vi "Compile Directional Speed 1.0 Data.vi"(8 "error in (no error)":errorcluster, 11 "Device Item Ref in":T3 format="%.0x") -> (0 "error out":errorcluster, 1 "bitfile names":string[](array[string]), 2 "Directional Speeds":T1[](array[typedef]), 3 "Device Item Ref out":T3 format="%.0x")   [LabVIEW 2015, in "Engine Simulation Toolkit System Explorer.lvlib"]
uses:
  Engine Simulation Toolkit System Explorer.lvlib
  <vilib>/NI Veristand/Custom Device API/Custom Device Item Ref.ctl
  Shared/1.0 Directional Speed Engine Data.ctl
  Shared/1.0 Directional Speed FIFO Idxs.ctl
  Digital Pattern Find Events Enum.ctl
  Custom wrapped 10 bit counter.vi
  Shared/Constants and GUIDs.vi
  <vilib>/NI Veristand/Custom Device Tools/Custom Device Utility Library/NI VeriStand - Search for All Items by GUID.vi
  Shared/Properties.vi
  <vilib>/NI Veristand/Custom Device API/Get Item Property (String).vi
  <vilib>/NI Veristand/Custom Device API/Get Item Property (Dependent Node Pointer).vi
  <vilib>/NI Veristand/Custom Device Tools/Custom Device Utility Library/Custom Device Utility Library.lvlib
  Shared/Engine Simulation Toolkit Shared.lvlib
  <vilib>/NI Veristand/Custom Device API/Custom Device API.lvlib
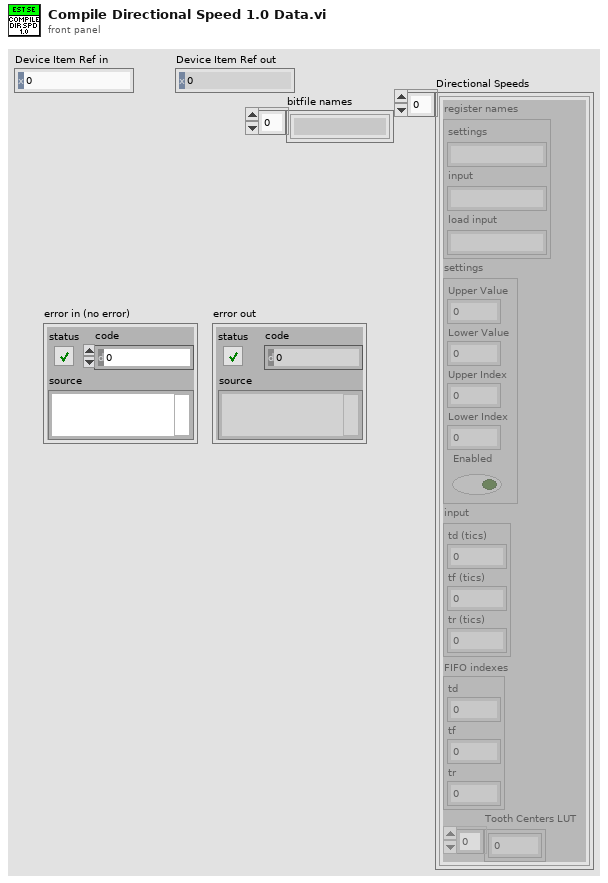
[diagram p1: front panel]
types:
  T1 = typedef "Engine Simulation Toolkit Shared.lvlib/1.0 Directional Speed Engine Data.ctl" = cluster{"register names":cluster{"settings":string, "input":string, "load input":string}, "settings":cluster{"Upper Value":u16, "Lower Value":u16, "Upper Index":fxp<+,10,10>, "Lower Index":fxp<+,10,10>, "Enabled":bool}, "input":cluster{"td (tics)":u16, "tf (tics)":u16, "tr (tics)":u16}, "FIFO indexes":T2, "Tooth Centers LUT":u16[]}
  T2 = typedef "Engine Simulation Toolkit Shared.lvlib/1.0 Directional Speed FIFO Idxs.ctl" = cluster{"td":i32, "tf":i32, "tr":i32}
  T3 = typedef "Custom Device API.lvlib/Custom Device Item Ref.ctl" = u64
  T4 = typedef "Engine Simulation Toolkit Shared.lvlib/Channel.ctl" = cluster{"Name":string, "Units":string, "Default":dbl, "Description":string}
  T5 = typedef "Engine Simulation Toolkit System Explorer.lvlib/Digital Pattern Find Events Enum.ctl" = enum16{"Rising Edge", "Falling Edge", "Any Edge", "Center Tooth", "Center Gap"}
  T6 = typedef "Custom Device API.lvlib/Custom Device Item Info.ctl" = cluster{"Name":string, "Is Channel":bool, "GUID":string, "Is Waveform":bool}
  T7 = typedef "Engine Simulation Toolkit System Explorer.lvlib/Digital Pattern.ctl" = cluster{"Name":string, "Base":T8, "Remove":T9[], "Add":T10[], "FPGA Resource":string}
  T8 = typedef "Engine Simulation Toolkit System Explorer.lvlib/Digital Pattern Base.ctl" = cluster{"Length":dbl, "Teeth":u16, "Width":dbl, "Offset":dbl}
  T9 = typedef "Engine Simulation Toolkit System Explorer.lvlib/Digital Pattern Remove Edge.ctl" = cluster{"Tooth":u16, "Edge":bool}
  T10 = typedef "Engine Simulation Toolkit System Explorer.lvlib/Digital Pattern Add Pulse.ctl" = cluster{"Tooth":u16, "Offset":dbl, "Width":dbl}
  T11 = typedef "Engine Simulation Toolkit System Explorer.lvlib/Digital Pattern Expanded.ctl" = cluster{"X":dbl[], "Y":dbl[]}
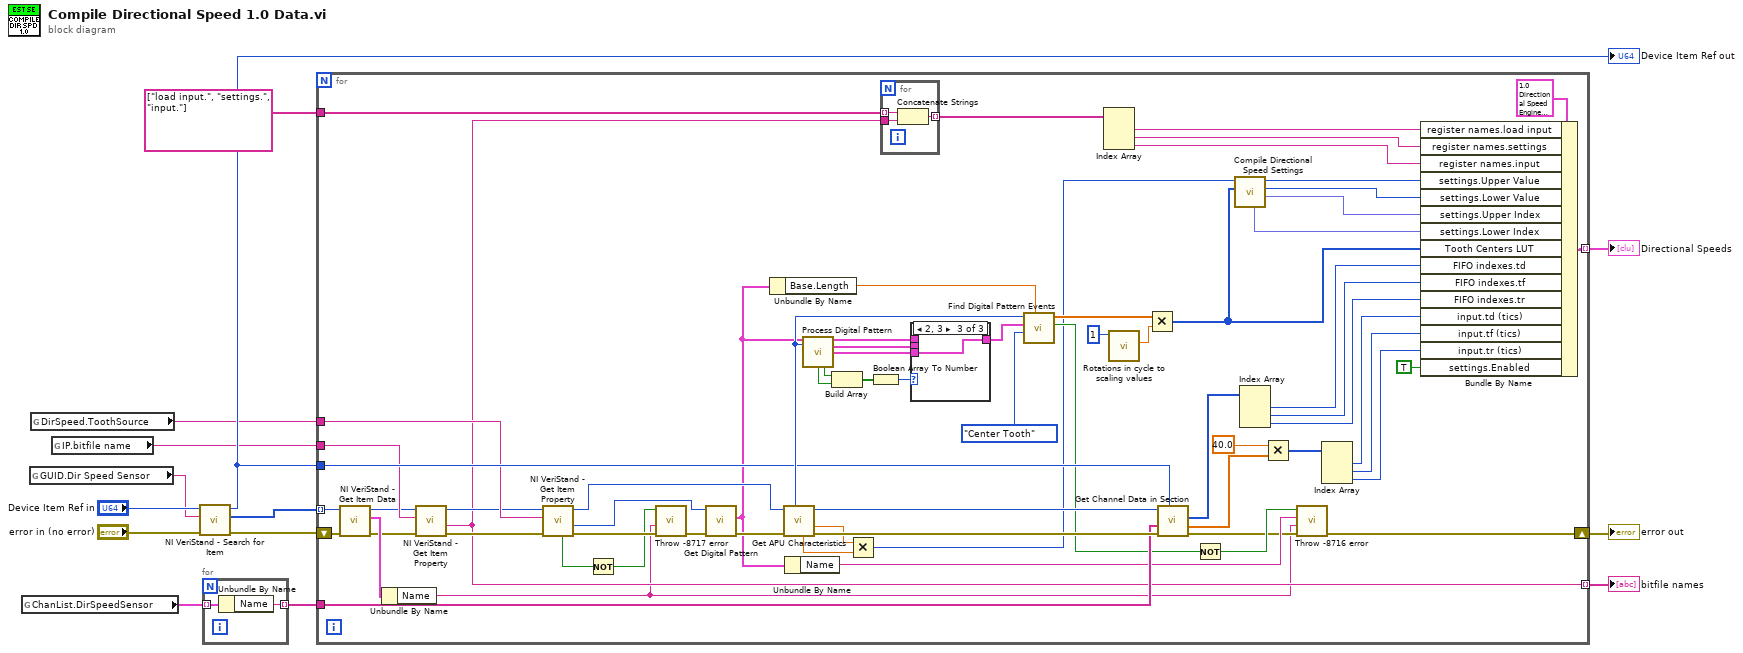
[diagram p0: block diagram]
diagram:
  n1 = global read "Constants and GUIDs.vi" "ChanList.DirSpeedSensor"() -> (w6:T4[])
  n2 = global read "Constants and GUIDs.vi" "GUID.Dir Speed Sensor"() -> (w12:string)
  n3 = global read "Properties.vi" "DirSpeed.ToothSource"() -> (w4:string)
  n4 = global read "Properties.vi" "IP.bitfile name"() -> (w3:string)
  n5 = call-poly <vilib>:"NI VeriStand - Search for Item.vi"("error in"="error in (no error)", "Item GUID"=w12, "Section Ref in"="Device Item Ref in") -> ("error out"=w11:errorcluster, "Item Refs"=w7:T3[], "Section Ref out"=w8:T3)  [unwired: 5 in, 1 out]
  "Device Item Ref out" <- w8
  n6 = for {
    tunnel: [w16] -> w5 mode=indexing
    tunnel: w6 -> [w15] mode=indexing
    n7 = Unbundle By Name(w15) -> ("Name"=w16:string)
  }
  n8 = for {
    shift-right: [w48] -> w9
    shift-left: w11 -> [w41]
    tunnel: string[] ["load input.", "settings.", "input."] -> [w54]
    tunnel: [w81] -> w1 mode=indexing
    tunnel: w8 -> [w73]
    tunnel: w7 -> [w38] mode=indexing
    tunnel: w5 -> [w72]
    tunnel: w4 -> [w59]
    tunnel: w3 -> [w50]
    tunnel: [w49] -> w2 mode=indexing
    n9 = call <vilib>:"NI VeriStand - Get Item Data.vi"("error in (no error)"=w41, "Item Ref in"=w38) -> ("error out"=w40:errorcluster, "Item Info"=w43:T6, "Item Ref out"=w39:T3)  [unwired: 6 in, 1 out]
    n10 = Unbundle By Name(w43) -> ("Name"=w34:string)
    n11 = call-poly <vilib>:"NI VeriStand - Get Item Property.vi"("error in (no error)"=w40, "Property Name"=w50, "Item Ref in"=w39) -> ("error out"=w52:errorcluster, "Value"=w49:string, "Item Ref out"=w51:T3)  [unwired: 5 in, 1 out]
    n12 = call-poly <vilib>:"NI VeriStand - Get Item Property.vi"("error in (no error)"=w52, "Property Name"=w59, "Item Ref in"=w51) -> ("error out"=w60:errorcluster, "Dependent Node Ref"=w57:T3, "Item Ref out"=w56:T3, "Found"=w36:bool)  [unwired: 5 in]
    n13 = Not(x=w36) -> (.not. x?=w35:bool)
    n14 = call "Throw -8717 error.vi"("error in (no error)"=w60, "dir speed name"=w34, "error"=w35) -> ("error out"=w37:errorcluster)  [unwired: 8 in]
    n15 = call "Get Digital Pattern.vi"("error in (no error)"=w37, "Item Ref in"=w57) -> ("error out"=w58:errorcluster, "EPT Pattern"=w45:T7)  [unwired: 7 in, 1 out]
    n16 = Unbundle By Name(w45) -> ("Base.Length"=w77:dbl)
    n17 = call "Get APU Characteristics.vi"("error in (no error)"=w58, "Item Ref in"=w56) -> ("error out"=w75:errorcluster, "angle to u16 scale factor"=w33:dbl, "Item Ref out"=w55:T3, "start angle"=w32:dbl, "rotations"=w78:u16)  [unwired: 3 in, 2 out]
    n18 = Unbundle By Name(w45) -> ("Name"=w44:string)
    n19 = call "Process Digital Pattern.vi"("EPT Pattern"=w45, "Rotations"=w78) -> ("Base"=w64:T11, 6:"Reduced"=w63:T11, 8:"Final"=w62:T11, 13:"Final"=w67:bool, 14:"Reduced"=w68:bool)  [unwired: 7 in, 2 out]
    n20 = Build Array(w68, w67) -> (w66:bool[])
    n21 = Multiply(x=w33, y=w32) -> (x*y=w31:u16)
    n22 = Boolean Array To Number(Boolean array=w66) -> (number=w65:u32)
    n23 = for {
      tunnel: w49 -> [w87]
      tunnel: w54 -> [w86] mode=indexing
      tunnel: [w85] -> w53 mode=indexing
      n24 = Concatenate Strings(w86, w87) -> (w85:string)
    }
    n25 = case shown="2, 3" w65 {
      tunnel: w64 -> [w88 _ _]
      tunnel: w63 -> [_ w89 _]
      tunnel: w62 -> [_ _ w90]
      tunnel: [w88 w89 w90] -> w61
      frame 0, Default {
      }
      frame 1 {
      }
      frame 2, 3 {
      }
    }
    n26 = call "Find Digital Pattern Events.vi"("Base.length"=w77, "Event"=Digital_Pattern_Find_Events_Enum."Center Tooth", "Pattern"=w61, "Rotations"=w78) -> ("crank angle"=w47:bool, "Locations"=w74:dbl[])  [unwired: 5 in, 1 out]
    n27 = Index Array(array=w53) -> (element #1=w83:string, element #2=w82:string, element #3=w80:string)  [unwired: 3 in]
    n28 = call "Rotations in cycle to scaling values.vi"("rotations in a cycle"=u16 1) -> ("angle to u16 scale factor"=w69:dbl)  [unwired: 8 in, 2 out]
    n29 = Multiply(x=w74, y=w69) -> (x*y=w26:u16[])
    n30 = call "Get Channel Data in Section.vi"("Custom device ref"=w73, "error in (no error)"=w75, "Channels"=w72, "Item Ref in"=w55) -> ("error out"=w42:errorcluster, "default values"=w70:dbl[], "FIFO indexes"=w71:i32[])  [unwired: 3 in, 2 out]
    n31 = Not(x=w47) -> (.not. x?=w46:bool)
    n32 = call "Compile Directional Speed Settings.vi"("Tooth centers"=w26, "APU start position"=w31) -> ("upper index"=w28:fxp<+,10,10>, "lower value"=w29:u16, "upper value"=w30:u16, "lower index"=w27:fxp<+,10,10>)  [unwired: 6 in]
    n33 = Index Array(array=w71) -> (element #1=w25:i32, element #2=w24:i32, element #3=w23:i32)  [unwired: 3 in]
    n34 = Multiply(x=40.0 ("rotations in a cycle"), y=w70) -> (x*y=w22:u16[])
    n35 = call "Throw -8716 error.vi"("error in (no error)"=w42, "dir speed name"=w34, "tooth source name"=w44, "error"=w46) -> ("error out"=w48:errorcluster)  [unwired: 7 in]
    n36 = Index Array(array=w22) -> (element #1=w20:u16, element #2=w19:u16, element #3=w18:u16)  [unwired: 3 in]
    n37 = Bundle By Name(cluster=T1 {"register names"={"settings"="", "input"="", "load input"=""}, "settings"={"Upper Value"=0, "Lower Value"=0, "Upper Index"=0.0, "Lower Index"=0.0, "Enabled"=FALSE}, "input"={"td (tics)"=0, "tf (tics)"=0, "tr (tics)"=0}, "FIFO indexes"={"td"=0, "tf"=0, "tr"=0}, "Tooth Centers LUT"=[]} ("1.0.0 Directional Speed"), "register names.load input"=w83, "register names.settings"=w82, "register names.input"=w80, "settings.Upper Value"=w30, "settings.Lower Value"=w29, "settings.Upper Index"=w28, "settings.Lower Index"=w27, "Tooth Centers LUT"=w26, "FIFO indexes.td"=w25, "FIFO indexes.tf"=w24, "FIFO indexes.tr"=w23, "input.td (tics)"=w20, "input.tf (tics)"=w19, "input.tr (tics)"=w18, "settings.Enabled"=TRUE) -> (w81:T1)
  }
  "error out" <- w9
  "Directional Speeds" <- w1
  "bitfile names" <- w2
